vi "_Serial_Mark10-Setup.vi"(5 "Serial Port":refnum<visa-resource-name>="COM5") -> (2 "VISA resource name out":refnum<visa-resource-name>)   [LabVIEW 2015]
panel:
  # "MARK10 Gauge Setup"
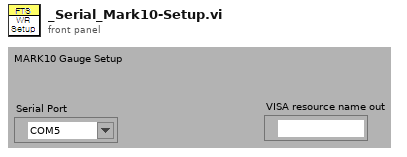
[diagram p1: front panel]
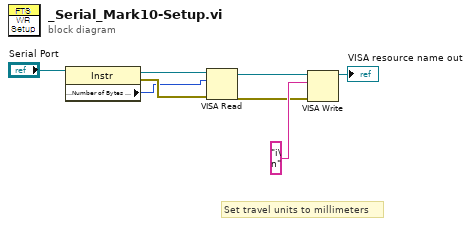
[diagram p0: block diagram]
diagram:
  # "Set travel units to millimeters"
  n1 = property class="Instr"(reference="Serial Port") -> (reference out=w7:refnum<visa-resource-name>, error out=w5:errorcluster, "Serial Settings:Number of Bytes at Serial Port"=w2:u32)  [unwired: 1 in]
  n2 = VISA Read(VISA resource name=w7, byte count=w2, error in (no error)=w5) -> (VISA resource name out=w4:refnum<visa-resource-name>, error out=w3:errorcluster)  [unwired: 2 out]
  n3 = VISA Write(VISA resource name=w4, write buffer="i\n", error in (no error)=w3) -> (VISA resource name out=→"VISA resource name out":refnum<visa-resource-name>)  [unwired: 2 out]
